vi "Get VIHostInterop Assembly Path.vi"() -> (3 "VIHost.Interop Assembly":path=path "NationalInstruments.VIHost.Interop.dll")   [LabVIEW 2021, in "InstrumentStudio Plugin SDK.lvlib" / "Plugin Session.lvclass"]
uses:
  Plugin Session.lvclass
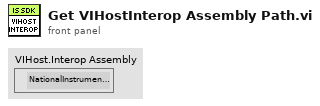
[diagram p1: front panel]
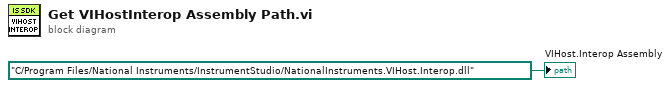
[diagram p0: block diagram]
diagram:
  "VIHost.Interop Assembly" <- path "C:/Program Files/National Instruments/InstrumentStudio/NationalInstruments.VIHost.Interop.dll" ("path in")
